vi "RT Loop - UI Commands.vi"(11 "Message Queue":refnum<queue>) -> ()   [LabVIEW 2020]
doc: "Use this template to build a simple state machine design pattern. Each state executes code and determines which state to transition to."
uses:
  support/Message Queue/Message Cluster.ctl
  controls/RT Loop - UI Communication State.ctl
  Globals/Global - Configuration Options.vi
  Globals/Global - All RT Loop Stop.vi
  Globals/Global - RT Stream Connections.vi
  support/Message Queue/Message Queue.lvlib
  <resource>/objmgr/ni.dex.rc
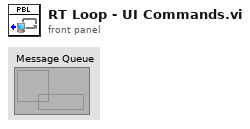
[diagram p1: front panel]
types:
  T1 = typedef "RT Loop - UI Communication State.ctl" = enum16{"Initialize", "Listen for UI Writer", "Receive UI Commands"}
  T2 = typedef "Message Queue.lvlib/Message Cluster.ctl" = cluster{"Message":string, "Message Data":variant}
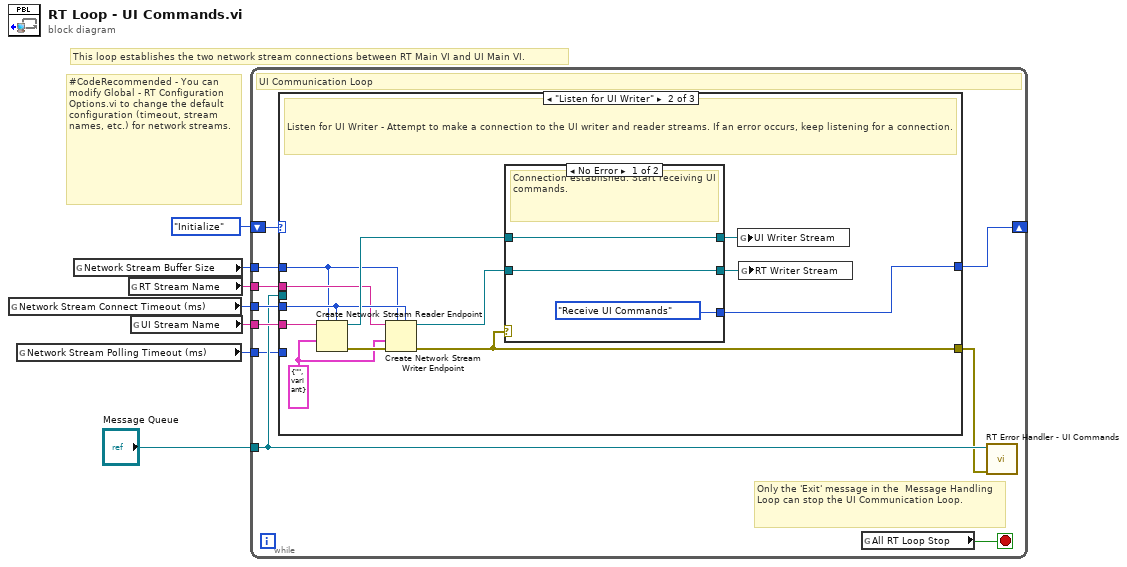
[diagram p0: block diagram]
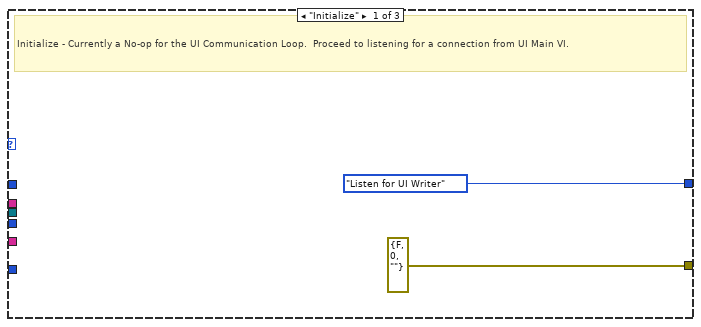
[diagram p2: hidden frame]
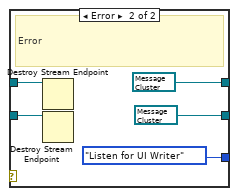
[diagram p3: hidden frame]
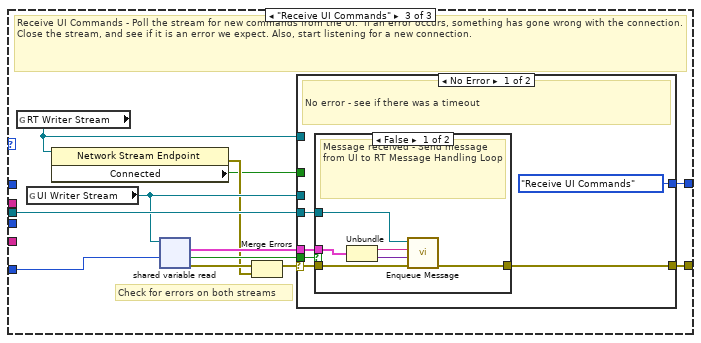
[diagram p4: hidden frame]
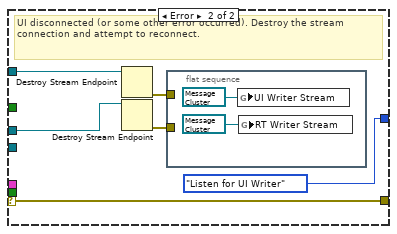
[diagram p6: hidden frame]
diagram:
  # "#CodeRecommended - You can modify Global - RT Configuration Options.vi to change the default configuration (timeout, stream names, etc.) for network streams."
  # "This loop establishes the two network stream connections between RT Main VI and UI Main VI."
  n1 = global read "Global - Configuration Options.vi" "Network Stream Connect Timeout (ms)"() -> (w5:i32)
  n2 = global read "Global - Configuration Options.vi" "Network Stream Polling Timeout (ms)"() -> (w2:i32)
  n3 = global read "Global - Configuration Options.vi" "Network Stream Buffer Size"() -> (w1:i32)
  n4 = global read "Global - Configuration Options.vi" "RT Stream Name"() -> (w3:string)
  n5 = global read "Global - Configuration Options.vi" "UI Stream Name"() -> (w4:string)
  n6 = while {
    shift-right: [w16] -> _
    shift-left: RT_Loop_-_UI_Communication_State."Initialize" ("RT Loop - Host Communication State") -> [w17]
    tunnel: "Message Queue" -> [w12]
    tunnel: w5 -> [w14]
    tunnel: w4 -> [w13]
    tunnel: w3 -> [w10]
    tunnel: w2 -> [w9]
    tunnel: w1 -> [w8]
    stop <- w15 stop-if-true
    # "Only the 'Exit' message in the  Message Handling Loop can stop the UI Communication Loop."
    # "UI Communication Loop"
    n7 = case shown="\"Listen for UI Writer\"" w17 {
      tunnel: [RT_Loop_-_UI_Communication_State."Listen for UI Writer" ("RT Loop - Host Communication State") w30 w50] -> w16
      tunnel: [errorcluster {"status"=FALSE, "code"=0, "source"=""} ("error IO") w25 w51] -> w11
      tunnel: w14 -> [_ w24 _]
      tunnel: w13 -> [_ w29 _]
      tunnel: w12 -> [_ _ w49]
      tunnel: w10 -> [_ w23 _]
      tunnel: w9 -> [_ _ w40]
      tunnel: w8 -> [_ w20 _]
      frame "Initialize" {
        # "Initialize - Currently a No-op for the UI Communication Loop.  Proceed to listening for a connection from UI Main VI."
      }
      frame "Listen for UI Writer" {
        w27 = T2 {"Message"="", "Message Data"=variant} ("Message Cluster")
        # "Listen for UI Writer - Attempt to make a connection to the UI writer and reader streams. If an error occurs, keep listening for a connection."
        n8 = Create Network Stream Reader Endpoint(5:w24, 7:w20, 9:w27, 11:w29) -> (0:w28:errorcluster, 3:w31:refnum<k21>)  [unwired: 3 in]
        n9 = Create Network Stream Writer Endpoint(5:w24, 7:w20, 8:w28, 9:w27, 11:w23) -> (0:w25:errorcluster, 3:w26:refnum<k21>)  [unwired: 2 in]
        n10 = case shown="No Error" w25 {
          tunnel: w31 -> [w33 w36]
          tunnel: [RT_Loop_-_UI_Communication_State."Receive UI Commands" ("RT Loop - Host Communication State") RT_Loop_-_UI_Communication_State."Listen for UI Writer" ("RT Loop - Host Communication State")] -> w30
          tunnel: w26 -> [w32 w35]
          tunnel: [w33 refnum<k21> refnum] -> w22
          tunnel: [w32 refnum<k21> refnum] -> w21
          frame No Error {
            # "Connection established. Start receiving UI commands."
          }
          frame Error {
            # "Error"
            n11 = Destroy Stream Endpoint(11:w36) -> ()  [unwired: 1 in, 1 out]
            n12 = Destroy Stream Endpoint(11:w35) -> ()  [unwired: 1 in, 1 out]
          }
        }
        n13 = global write "Global - RT Stream Connections.vi" "UI Writer Stream"(w22) -> ()
        n14 = global write "Global - RT Stream Connections.vi" "RT Writer Stream"(w21) -> ()
      }
      frame "Receive UI Commands" {
        # "Check for errors on both streams"
        # "Receive UI Commands - Poll the stream for new commands from the UI.  If an error occurs, something has gone wrong with the connection. Close the stream, and see if it is an error we expect. Also, start listening for a new connection."
        n15 = global read "Global - RT Stream Connections.vi" "RT Writer Stream"() -> (w41:refnum<k21>)
        n16 = global read "Global - RT Stream Connections.vi" "UI Writer Stream"() -> (w45:refnum<k21>)
        n17 = property class="Network Stream Endpoint"(reference=w41) -> (error out=w43:errorcluster, "Connected"=w42:bool)  [unwired: 1 in, 1 out]
        n18 = shared-variable-read(w45, w40) -> (w46:errorcluster, w47:bool, w48:T2)  [unwired: 1 in, 1 out]
        n19 = Merge Errors(w46, w43) -> (w44:errorcluster)
        n20 = case shown="No Error" w44 {
          selector: w44 -> [w55 w69]
          tunnel: [w54 w69] -> w51
          tunnel: w47 -> [w57 _]
          tunnel: w48 -> [w56 _]
          tunnel: [RT_Loop_-_UI_Communication_State."Receive UI Commands" ("RT Loop - Host Communication State") RT_Loop_-_UI_Communication_State."Listen for UI Writer" ("RT Loop - Host Communication State")] -> w50
          tunnel: w49 -> [w53 _]
          tunnel: w45 -> [_ w66]
          tunnel: w42 -> [_ _]
          tunnel: w41 -> [_ w65]
          frame No Error {
            # "No error - see if there was a timeout"
            n21 = case shown="False" w57 {
              tunnel: w56 -> [w62 _]
              tunnel: w55 -> [w63 w64]
              tunnel: [w58 w64] -> w54
              tunnel: w53 -> [w59 _]
              frame False {
                # "Message received - Send message from UI to RT Message Handling Loop"
                n22 = Unbundle(w62) -> ("Message"=w61:string, "Message Data"=w60:variant)
                n23 = call "Enqueue Message.vi"("error in (no error)"=w63, "Message Data"=w60, "Message"=w61, "Message Queue"=w59) -> ("error out"=w58:errorcluster)  [unwired: 6 in, 1 out]
              }
              frame True {
                # "Timeout - no new command"
              }
            }
          }
          frame Error {
            # "UI disconnected (or some other error occurred). Destroy the stream connection and attempt to reconnect."
            n24 = Destroy Stream Endpoint(11:w65) -> (0:w68:errorcluster)  [unwired: 1 in]
            n25 = Destroy Stream Endpoint(11:w66) -> (0:w67:errorcluster)  [unwired: 1 in]
            n26 = flat-sequence {
              tunnel: w68 -> [_]
              tunnel: w67 -> [_]
              frame #0 {
                n27 = global write "Global - RT Stream Connections.vi" "UI Writer Stream"(refnum<k21> refnum ("Host Writer Stream")) -> ()
                n28 = global write "Global - RT Stream Connections.vi" "RT Writer Stream"(refnum<k21> refnum ("RT Writer Stream")) -> ()
              }
            }
          }
        }
      }
    }
    n29 = global read "Global - All RT Loop Stop.vi" "All RT Loop Stop"() -> (w15:bool)
    n30 = call "RT Error Handler - UI Commands.vi"("error in (no error)"=w11, "Message Queue"=w12) -> ()  [unwired: 9 in, 1 out]
  }
